vi "Initialize.vi"(8 "error in":errorcluster, 10 "shared resources":refnum<class "Shared Resources.lvclass">, 11 "logging execution unit in":refnum<class "Logging Execution Unit.lvclass">) -> (0 "error out":errorcluster, 3 "logging execution unit out":refnum<class "Logging Execution Unit.lvclass">)   [LabVIEW 2020, in "Ballard MIL-STD-1553 Engine.lvlib" / "Implementation.lvlib" / "Logging Execution Unit.lvclass"]
uses:
  Logging Execution Unit.lvclass
  C:/Users/nitest/Desktop/Git 2020/niveristand-aim-milStd1553-custom-device/Source/Custom Device Support/Engine/Implementation/Execution Unit/Execution Unit.lvclass
  Interfaces/Shared Resources/Shared Resources.lvclass
  Shared Resources/Shared Resources.lvclass
  Logging Execution Unit.lvclass/Logging Execution Unit.ctl
  Execution Unit/Execution Unit.lvclass/Execution Unit.ctl
  Execution Unit/Execution Unit.lvclass
  <instrlib>/BTICardLib/BTICardLV.lvlib
  C:/Users/nitest/Desktop/Git 2020/niveristand-aim-milStd1553-custom-device/Source/Custom Device Support/Engine/Interfaces/Execution Unit/Execution Unit.lvclass
  C:/Users/nitest/Desktop/Git 2020/niveristand-aim-milStd1553-custom-device/Source/Custom Device Support/Engine/Implementation/Logging Execution Unit/Logging Execution Unit.lvclass
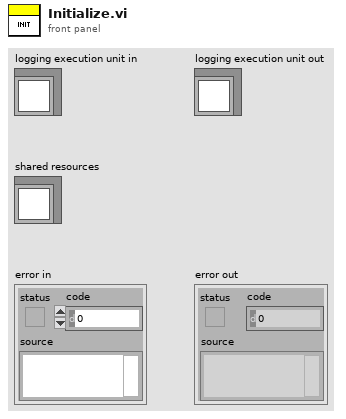
[diagram p1: front panel]
types:
  T1 = typedef "Ballard MIL-STD-1553 Engine.lvlib/Custom Device.lvlib/Hardware Handles.ctl" = cluster{"core handle":u64, "core reader handle":u64, "channel handles":u64[]}
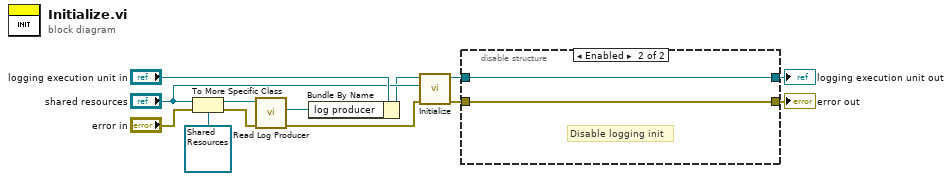
[diagram p0: block diagram]
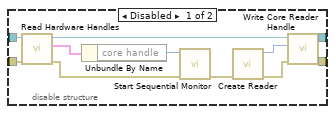
[diagram p2: hidden frame]
diagram:
  n1 = To More Specific Class(target class=refnum<class "Shared Resources.lvclass"> refnum ("Shared Resources in"), reference="shared resources", error in="error in") -> (specific class reference=w6:refnum<class "Shared Resources.lvclass">, error out=w11:errorcluster)
  n2 = call-dynamic "Read Log Producer.vi"("error in (no error)"=w11, "Shared Resources in"=w6) -> ("error out"=w13:errorcluster, "Communication Bus Template Interfaces:Implementation.lvlib:Word Logging.lvlib:Log Producer.lvclass"=w9:refnum<class "Log Producer.lvclass">)  [unwired: 7 in, 1 out]
  n3 = Bundle By Name(cluster="logging execution unit in", "log producer"=w9) -> (w1:refnum<class "Logging Execution Unit.lvclass">)
  n4 = call-parent "Initialize.vi"("error in"=w13, "shared resources"="shared resources", "Execution Unit Implementation in"=w1) -> ("error out"=w4:errorcluster, "Execution Unit Implementation out"=w5:refnum<class "Logging Execution Unit.lvclass">)  [unwired: 7 in]
  n5 = disable-structure shown="Enabled" {
    disable-tunnel: w5 -> [w23 w26]
    disable-tunnel: w4 -> [w22 w25]
    disable-tunnel: [w18 w26] -> w3
    disable-tunnel: [w16 w25] -> w2
    frame Disabled {
      n6 = call "Read Hardware Handles.vi"("error in"=w22, "Execution Unit in"=w23) -> ("error out"=w19:errorcluster, "hardware handles"=w21:T1, "Execution Unit out"=w14:refnum<class "Logging Execution Unit.lvclass">)  [unwired: 7 in]
      n7 = Unbundle By Name(w21) -> ("core handle"=w20:u64)
      n8 = call <instrlib>:"Start Sequential Monitor.vi"("error in (no error)"=w19, "core handle in"=w20) -> ("error out"=w24:errorcluster)  [unwired: 8 in, 1 out]
      n9 = call <instrlib>:"Create Reader.vi"("error in (no error)"=w24) -> ("error out"=w17:errorcluster, "core reader handle out"=w15:u64)  [unwired: 9 in]
      n10 = call "Write Core Reader Handle.vi"("error in"=w17, "core reader handle"=w15, "execution unit in"=w14) -> ("error out"=w16:errorcluster, "execution unit out"=w18:refnum<class "Logging Execution Unit.lvclass">)  [unwired: 7 in]
    }
    frame Enabled {
      # "Disable logging init"
    }
  }
  "error out" <- w2
  "logging execution unit out" <- w3
